vi "MHTML Base64.vi"(7 "Binary String":string) -> (8 "String (Base64)":string)   [LabVIEW 2011]
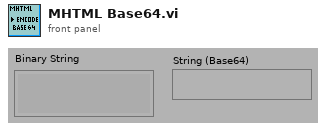
[diagram p1: front panel]
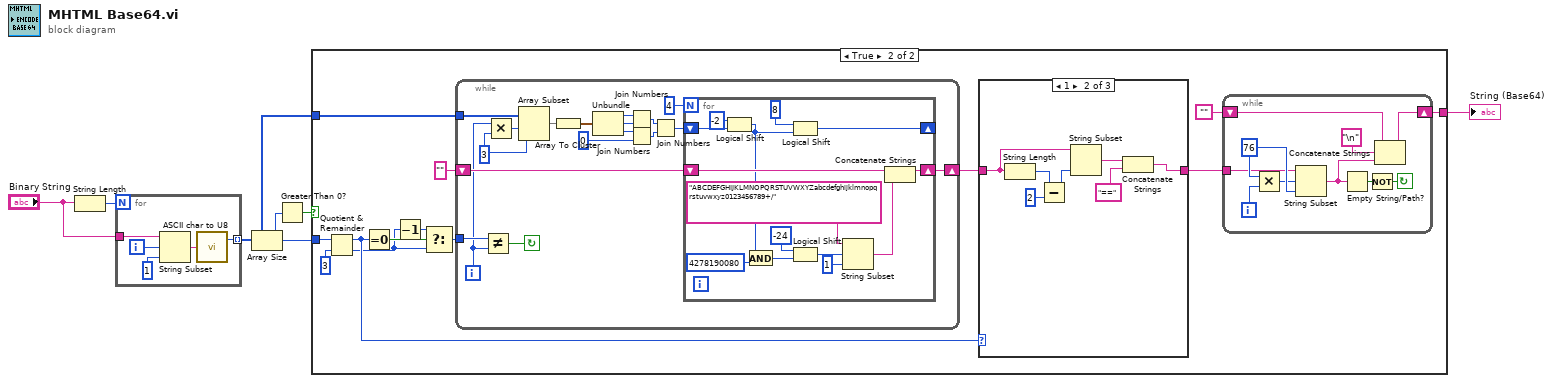
[diagram p0: block diagram]
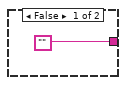
[diagram p2: hidden frame]
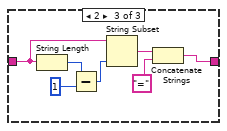
[diagram p4: hidden frame]
diagram:
  n1 = String Length(string="Binary String") -> (length=w3:i32)
  n2 = for {
    N: w3 -> [_]
    tunnel: "Binary String" -> [w11]
    tunnel: [w7] -> w1 mode=indexing
    i -> [w10]
    n3 = String Subset(string=w11, offset (0)=w10, length (rest)=1 ("length")) -> (substring=w8:string)
    n4 = call "ASCII char to U8.vi"("ASCII character(s)"=w8) -> ("first ASCII value (U8)"=w7:u8)  [unwired: 1 out]
  }
  n5 = Array Size(array=w1) -> (size(s)=w6:i32)
  n6 = Greater Than 0?(x=w6) -> (x > 0?=w2:bool)
  n7 = case shown="True" w2 {
    tunnel: w6 -> [_ w24]
    tunnel: ["" w16] -> w5
    tunnel: w1 -> [_ w15]
    frame False {
    }
    frame True {
      n8 = Quotient & Remainder(x=w24, y=3) -> (x-y*floor(x/y)=w22:i32, floor(x/y)=w19:i32)
      n9 = Equal To 0?(x=w22) -> (x = 0?=w21:bool)
      n10 = Decrement(x=w19) -> (x-1=w18:i32)
      n11 = Select(t=w18, s=w21, f=w19) -> (s? t:f=w20:i32)
      n12 = while {
        tunnel: w20 -> [w29]
        shift-left: "" -> [w32]
        shift-right: [w31] -> w13
        tunnel: w15 -> [w43]
        i -> [w26]
        stop <- w28 continue-if-true
        w27 = 3 ("x")
        n13 = Not Equal?(x=w29, y=w26) -> (x != y?=w28:bool)
        n14 = Multiply(x=w26, y=w27) -> (x*y=w42:i32)
        n15 = Array Subset(array=w43, index=w42, length=w27) -> (w41:u8[])
        n16 = Array To Cluster(array=w41) -> (cluster=w40:cluster{"[0]":u8, "[1]":u8, "[2]":u8})
        n17 = Unbundle(w40) -> ("[0]"=w39:u8, "[1]"=w38:u8, "[2]"=w37:u8)
        n18 = Join Numbers(hi=w39, lo=w38) -> ((hi.lo)=w35:u16)
        n19 = Join Numbers(hi=w37, lo=u8 0) -> ((hi.lo)=w34:u16)
        n20 = Join Numbers(hi=w35, lo=w34) -> ((hi.lo)=w30:u32)
        n21 = for {
          N: 4 -> [_]
          shift-right: [w55] -> _
          shift-left: w30 -> [w57]
          shift-right: [w47] -> w31
          shift-left: w32 -> [w48]
          n22 = Logical Shift(y=i8 -2, x=w57) -> (x << y=w44:u32)
          n23 = And(x=w44, y=u32 4278190080) -> (x .and. y?=w46:u32)
          n24 = Logical Shift(y=i8 8, x=w44) -> (x << y=w55:u32)
          n25 = Logical Shift(y=i8 -24, x=w46) -> (x << y=w45:u32)
          n26 = String Subset(string="ABCDEFGHIJKLMNOPQRSTUVWXYZabcdefghijklmnopqrstuvwxyz0123456789+/", offset (0)=w45, length (rest)=1 ("length")) -> (substring=w49:string)
          n27 = Concatenate Strings(w48, w49) -> (w47:string)
        }
      }
      n28 = case shown="1" w22 {
        tunnel: w13 -> [w68 w75 w82]
        tunnel: [w68 w71 w78] -> w17
        frame 0, Default {
        }
        frame 1 {
          n29 = String Length(string=w75) -> (length=w73:i32)
          n30 = Subtract(x=w73, y=2) -> (x-y=w74:i32)
          n31 = String Subset(string=w75, length (rest)=w74) -> (substring=w72:string)  [unwired: 1 out]
          n32 = Concatenate Strings(w72, "==" ("Substring")) -> (w71:string)
        }
        frame 2 {
          n33 = String Length(string=w82) -> (length=w80:i32)
          n34 = Subtract(x=w80, y=1) -> (x-y=w81:i32)
          n35 = String Subset(string=w82, length (rest)=w81) -> (substring=w79:string)  [unwired: 1 out]
          n36 = Concatenate Strings(w79, "=" ("Substring")) -> (w78:string)
        }
      }
      n37 = while {
        tunnel: w17 -> [w58]
        shift-left: "" -> [w62]
        shift-right: [w61] -> w16
        i -> [w67]
        stop <- w63 continue-if-true
        w66 = 76 ("length")
        n38 = Multiply(x=w66, y=w67) -> (x*y=w65:i32)
        n39 = String Subset(string=w58, offset (0)=w65, length (rest)=w66) -> (substring=w60:string)
        n40 = Empty String/Path?(string/path=w60) -> (empty?=w64:bool)
        n41 = Not(x=w64) -> (.not. x?=w63:bool)
        n42 = Concatenate Strings(w62, "\n", w60) -> (w61:string)
      }
    }
  }
  "String (Base64)" <- w5
